vi "VISA_OPC.vi"(4 "OPC(T)":bool=TRUE, 8 "error in":errorcluster {"code" format="%.0x"}, 9 "Timeout":u32=30000, 11 "Session In":refnum<visa-resource-name>="GPIB0::4::INSTR") -> (0 "error out":errorcluster {"code" format="%.0x"}, 3 "Session Out":refnum<visa-resource-name>, 5 "OPC?(T)":bool)   [LabVIEW 2018]
doc: "Launches the Instrument I/O Assistant, which you can use to communicate with message-based instruments and graphically parse the response. For example you can communicate with an instrument that uses a serial, Ethernet, or GPIB interface."
panel:
  out "OPC?":dbl
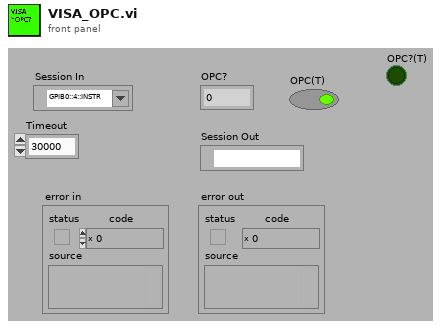
[diagram p1: front panel]
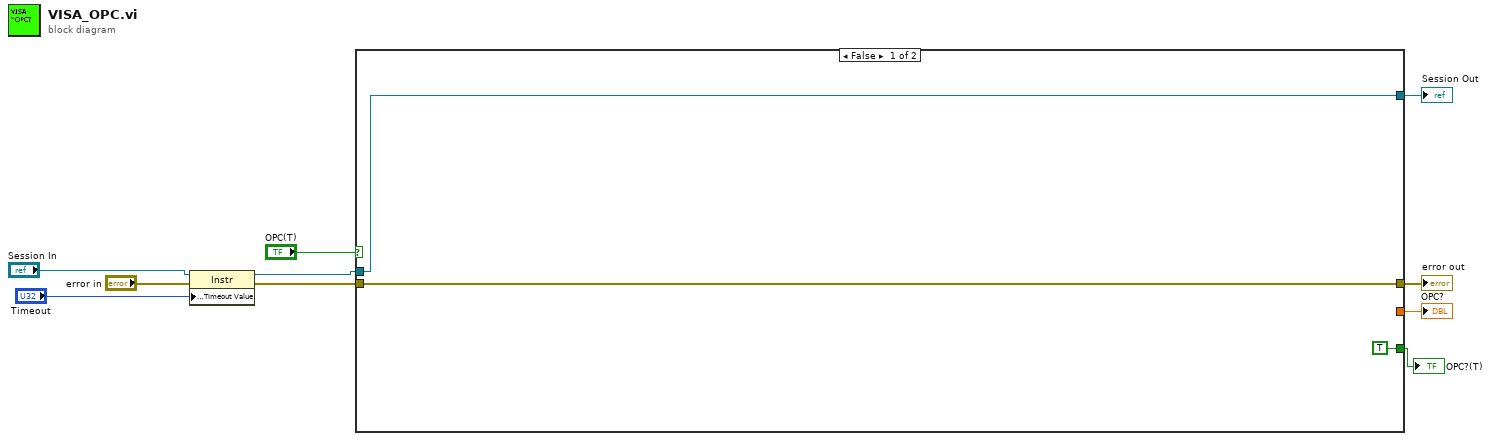
[diagram p0: block diagram]
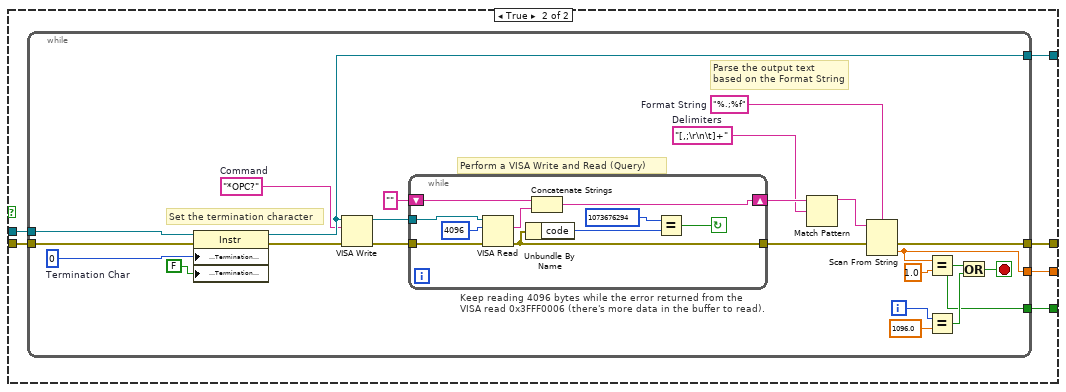
[diagram p2: hidden frame]
diagram:
  n1 = property class="Instr"(reference="Session In", error in="error in", "General Settings:Timeout Value"="Timeout") -> (reference out=w7:refnum<visa-resource-name>, error out=w6:errorcluster)
  n2 = case shown="False" "OPC(T)" {
    tunnel: w7 -> [w12 w19]
    tunnel: w6 -> [w13 w18]
    tunnel: [w12 w17] -> w5
    tunnel: [w13 w16] -> w4
    tunnel: [_ w15] -> w3
    tunnel: [TRUE w14] -> w1
    frame False {
    }
    frame True {
      n3 = while {
        tunnel: w19 -> [w42]
        tunnel: w18 -> [w41]
        tunnel: [w38] -> w17
        tunnel: [w28] -> w16
        tunnel: [w24] -> w15
        tunnel: [w20] -> w14
        i -> [w21]
        stop <- w26 stop-if-true
        w27 = "[,;\r\n\t]+"  # Delimiters
        w29 = "%.;%f"  # Format String
        w31 = "*OPC?"  # Command
        w39 = u8 0  # Termination Char
        # "Parse the output text based on the Format String"
        # "Perform a VISA Write and Read (Query)"
        # "Keep reading 4096 bytes while the error returned from the\nVISA read 0x3FFF0006 (there's more data in the buffer to read)."
        # "Set the termination character"
        n4 = property class="Instr"(reference=w42, error in=w41, "Message Based Settings:Termination Character"=w39, "Message Based Settings:Termination Character Enable"=FALSE ("enable")) -> (reference out=w38:refnum<visa-resource-name>, error out=w40:errorcluster)
        n5 = VISA Write(VISA resource name=w38, write buffer=w31, error in (no error)=w40) -> (VISA resource name out=w36:refnum<visa-resource-name>, error out=w34:errorcluster)  [unwired: 1 out]
        n6 = while {
          tunnel: w36 -> [w49]
          shift-right: [w43] -> w35
          shift-left: "" -> [w48]
          tunnel: w34 -> [w46]
          tunnel: [w45] -> w33
          stop <- w44 continue-if-true
          n7 = VISA Read(VISA resource name=w49, byte count=u32 4096 ("byte count (0)"), error in (no error)=w46) -> (read buffer=w47:string, error out=w45:errorcluster)  [unwired: 2 out]
          n8 = Unbundle By Name(w45) -> ("code"=w51:i32)
          n9 = Concatenate Strings(w48, w47) -> (w43:string)
          n10 = Equal?(x=1073676294, y=w51) -> (x = y?=w44:bool)
        }
        n11 = Match Pattern(string=w35, regular expression=w27) -> (before substring=w30:string)  [unwired: 1 in, 3 out]
        n12 = Scan From String(format string=w29, input string=w30, error in=w33) -> (error out=w28:errorcluster, output 1=w24:dbl)  [unwired: 2 in, 2 out]
        n13 = Equal?(x=w24, y=1.0) -> (x = y?=w20:bool)
        n14 = Equal?(x=w21, y=1096.0) -> (x = y?=w23:bool)
        n15 = Or(x=w20, y=w23) -> (x .or. y?=w26:bool)
      }
    }
  }
  "OPC?" <- w3
  "error out" <- w4
  "Session Out" <- w5
  "OPC?(T)" <- w1
